vi "Save Files.vi"(8 "error in":errorcluster, 10 "Write":bool, 11 "GUI Facade in":refnum<class "GUI Facade.lvclass">) -> (0 "error out":errorcluster, 3 "GUI Facade out":refnum<class "GUI Facade.lvclass">)   [LabVIEW 2018, in "GUI Facade.lvclass"]
uses:
  GUI Facade.lvclass
  File IO/Class/File Observer.lvclass
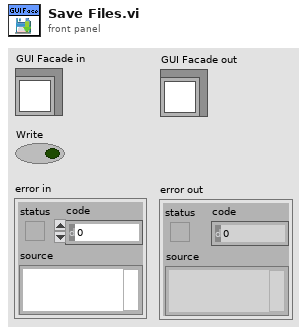
[diagram p1: front panel]
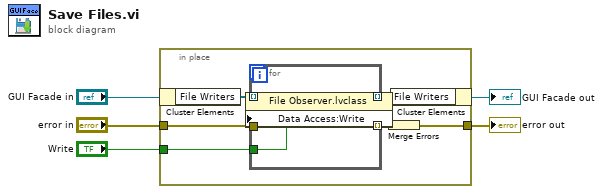
[diagram p0: block diagram]
diagram:
  n1 = in-place {
    in-place-border: "error in" -> [w9]
    in-place-border: [w7] -> w4
    in-place-border: "Write" -> [w6]
    n2 = in-place-cluster #1("GUI Facade in") -> ("File Writers"=w11:refnum<class "File Observer.lvclass">[])
    n3 = for {
      tunnel: w11 -> [w16] mode=indexing
      tunnel: [w15] -> w10 mode=indexing
      tunnel: w9 -> [w14]
      tunnel: [w13] -> w8 mode=indexing
      tunnel: w6 -> [w12]
      n4 = property class="File Observer.lvclass"(reference=w16, error in=w14, "Data Access:Write"=w12) -> (reference out=w15:refnum<class "File Observer.lvclass">, error out=w13:errorcluster)
    }
    n5 = Merge Errors(w8) -> (w7:errorcluster)
    n6 = in-place-cluster #1("File Writers"=w10) -> (→"GUI Facade out":refnum<class "GUI Facade.lvclass">)
  }
  "error out" <- w4
